vi "Lab5.vi"() -> ()   [LabVIEW 2011]
panel:
  out "XY Graph":cluster{dbl[], dbl[]}(graph)
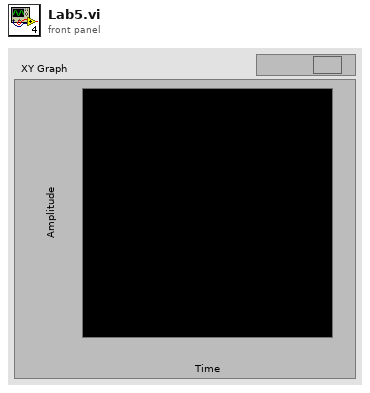
[diagram p1: front panel]
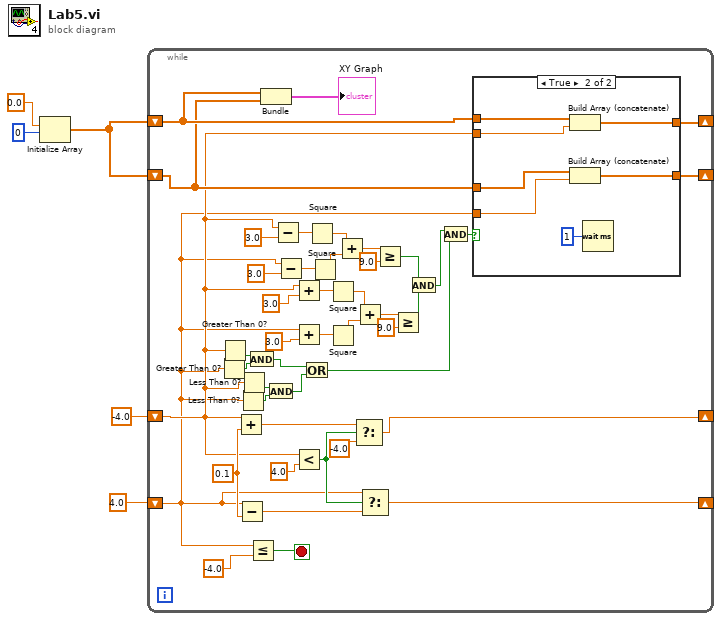
[diagram p0: block diagram]
diagram:
  n1 = Initialize Array(0.0 ("element"), 0 ("dimension size")) -> (w3:dbl[])
  n2 = while {
    shift-right: [w49] -> _
    shift-left: w3 -> [w46]
    shift-right: [w48] -> _
    shift-left: w3 -> [w45]
    shift-right: [w36] -> _
    shift-left: -4.0 ("element") -> [w12]
    shift-right: [w35] -> _
    shift-left: 4.0 ("element") -> [w11]
    stop <- w42 stop-if-true
    w44 = 0.1 ("y")
    n3 = Greater Than 0?(x=w11) -> (x > 0?=w15:bool)
    n4 = Greater Than 0?(x=w12) -> (x > 0?=w16:bool)
    n5 = Add(x=w12, y=w44) -> (x+y=w40:dbl)
    n6 = Subtract(x=w11, y=w44) -> (x-y=w39:dbl)
    n7 = Less Than 0?(x=w11) -> (x < 0?=w14:bool)
    n8 = Less Than 0?(x=w12) -> (x < 0?=w13:bool)
    n9 = And(x=w16, y=w15) -> (x .and. y?=w9:bool)
    n10 = Less Or Equal?(x=w11, y=-4.0 ("element")) -> (x <= y?=w42:bool)
    n11 = Bundle(w46, w45) -> (→"XY Graph":cluster{dbl[], dbl[]})  [unwired: 1 in]
    n12 = And(x=w13, y=w14) -> (x .and. y?=w10:bool)
    n13 = Subtract(x=w12, y=3.0) -> (x-y=w33:dbl)
    n14 = Subtract(x=w11, y=3.0) -> (x-y=w31:dbl)
    n15 = Add(x=w12, y=3.0) -> (x+y=w24:dbl)
    n16 = Add(x=w11, y=3.0) -> (x+y=w22:dbl)
    n17 = Less?(x=w12, y=4.0 ("element")) -> (x < y?=w37:bool)
    n18 = Or(x=w9, y=w10) -> (x .or. y?=w6:bool)
    n19 = Square(x=w33) -> (x^2=w30:dbl)
    n20 = Square(x=w31) -> (x^2=w29:dbl)
    n21 = Square(x=w24) -> (x^2=w21:dbl)
    n22 = Square(x=w22) -> (x^2=w20:dbl)
    n23 = Add(x=w30, y=w29) -> (x+y=w28:dbl)
    n24 = Select(t=w40, s=w37, f=-4.0 ("element")) -> (s? t:f=w36:dbl)
    n25 = Add(x=w21, y=w20) -> (x+y=w19:dbl)
    n26 = Select(t=w11, s=w37, f=w39) -> (s? t:f=w35:dbl)
    n27 = Greater Or Equal?(x=w28, y=9.0) -> (x >= y?=w26:bool)
    n28 = Greater Or Equal?(x=w19, y=9.0) -> (x >= y?=w17:bool)
    n29 = And(x=w26, y=w17) -> (x .and. y?=w7:bool)
    n30 = And(x=w7, y=w6) -> (x .and. y?=w8:bool)
    n31 = case shown="True" w8 {
      tunnel: [w51 w57] -> w49
      tunnel: [w50 w56] -> w48
      tunnel: w46 -> [w51 w55]
      tunnel: w45 -> [w50 w54]
      tunnel: w11 -> [_ w53]
      tunnel: w12 -> [_ w52]
      frame False {
      }
      frame True {
        n32 = Build Array (concatenate)(w55, w52) -> (w57:dbl[])
        n33 = Build Array (concatenate)(w54, w53) -> (w56:dbl[])
        n34 = Wait (ms)(milliseconds to wait=u32 1) -> ()  [unwired: 1 out]
      }
    }
  }
